vi "remove tag.vi"(8 "error in":errorcluster, 10 "tag":string, 11 "object ref in":T1) -> (0 "error out":errorcluster)   [LabVIEW 2013, in "Shared Memory Editor Node.lvclass"]
doc: "Copyright 2016 National Instruments Corporation\n\nLicensed under the Apache License, Version 2.0 (the \"License\"); you may not use this file except in compliance with the License. You may obtain a copy of the License at http://www.apache.org/licenses/LICENSE-2.0\nUnless required by applicable law or agreed to in writing, software distributed under the License is distributed on an \"AS IS\" BASIS, WITHOUT WARRANTIES OR CONDITIONS OF ANY KIND, either express or implied. See the License for the specific language governing permissions and limitations under the License."
uses:
  Shared Memory Editor Node.lvclass
  <vilib>/NI/DCAF Table API/Table Manager/object ref.ctl
  <vilib>/NI/DCAF/Tag Editor Core/Configuration Editor/Classes/Engine Parent/Engine Parent Editor Node.lvclass
  <vilib>/NI/DCAF/Tag Editor Core/Configuration Editor/Classes/Module editor node/module editor node.lvclass
  module/configuration/Shared Memory Configuration.lvclass
  <vilib>/NI/Configuration Framework/serializable configuration/NISE_CEF_serializable configuration.lvclass/NISE_CEF_serializable configuration.ctl
  <vilib>/Utility/LVClass/Get LV Class Name.vi
  <vilib>/NI/Configuration Framework/error generator/NISE_error generator.vi
  <vilib>/NI/Configuration Framework/serializable configuration/NISE_CEF_serializable configuration.lvclass
  <vilib>/NI/Module Execution Interface/Engine Configuration/engine configuration.lvclass
  <vilib>/NI/DCAF Table API/Table Manager/Table Manager.lvclass
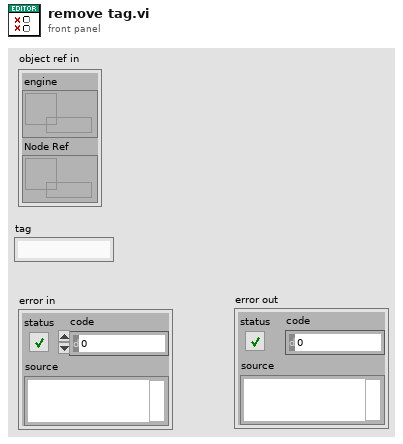
[diagram p1: front panel]
types:
  T1 = typedef "Table Manager.lvlib/Table Manager.lvclass/object ref.ctl" = cluster{"engine":refnum<data-value>, "Node Ref":refnum<data-value>}
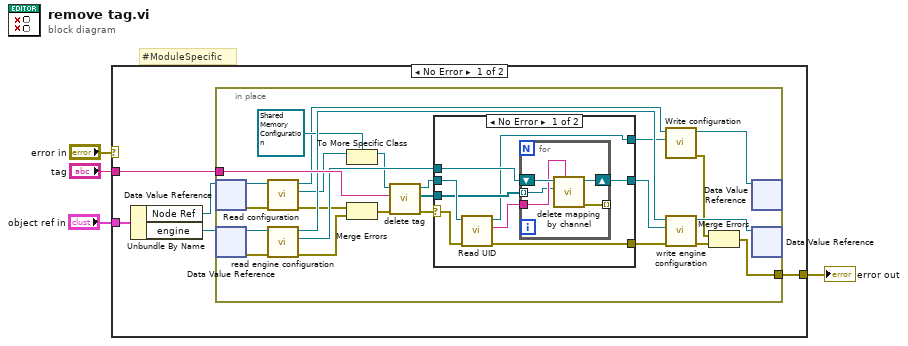
[diagram p0: block diagram]
diagram:
  # "#ModuleSpecific"
  n1 = case shown="No Error" "error in" {
    selector: "error in" -> [_ w51]
    tunnel: [w9 w51] -> w4
    tunnel: "object ref in" -> [w6 _]
    tunnel: "tag" -> [w5 _]
    frame No Error {
      n2 = Unbundle By Name(w6) -> ("Node Ref"=w7:refnum<data-value>, "engine"=w8:refnum<data-value>)
      n3 = in-place {
        in-place-border: [w10] -> w9
        in-place-border: w5 -> [w30]
        n4 = in-place-dvr #1(w7) -> (w29:refnum<class "module editor node.lvclass">, w31:errorcluster)
        n5 = in-place-dvr #2(w8) -> (w33:refnum<class "Engine Parent Editor Node.lvclass">, w32:errorcluster)
        n6 = call-dynamic "Read configuration.vi"("error in"=w31, "NISE_CEF_serializable node in"=w29) -> ("error out"=w15:errorcluster, "configuration"=w17:refnum<class "NISE_CEF_serializable configuration.lvclass">, "NISE_CEF_serializable node out"=w12:refnum<class "module editor node.lvclass">)  [unwired: 7 in]
        n7 = call <vilib>:"read engine configuration.vi"("error in"=w32, "Engine Parent Editor Node in"=w33) -> ("error out"=w24:errorcluster, "engine configuration"=w26:refnum<class "engine configuration.lvclass">, "Engine Parent Editor Node out"=w25:refnum<class "Engine Parent Editor Node.lvclass">)  [unwired: 7 in]
        n8 = To More Specific Class(target class=refnum<class "Shared Memory Configuration.lvclass"> refnum ("tag select  module configuration in"), reference=w17) -> (specific class reference=w16:refnum<class "Shared Memory Configuration.lvclass">)  [unwired: 1 in, 1 out]
        n9 = Merge Errors(w15, w24) -> (w23:errorcluster)
        n10 = call "delete tag.vi"("error in"=w23, "tag name"=w30, "shared memory module configuration"=w16) -> ("error out"=w22:errorcluster, "deleted channels"=w21:refnum<class "TBM channel.lvclass">[], "shared memory module configuration out"=w19:refnum<class "Shared Memory Configuration.lvclass">)  [unwired: 6 in]
        n11 = case shown="No Error" w22 {
          selector: w22 -> [w38 w49]
          tunnel: [w37 w49] -> w20
          tunnel: w19 -> [w40 w48]
          tunnel: w26 -> [w42 w50]
          tunnel: [w41 w50] -> w27
          tunnel: w21 -> [w36 _]
          tunnel: [w35 w48] -> w11
          frame No Error {
            n12 = call <vilib>:"Read UID.vi"("error in"=w38, "configuration in"=w40) -> ("error out"=w37:errorcluster, "instance id"=w39:string, "configuration out"=w35:refnum<class "Shared Memory Configuration.lvclass">)  [unwired: 7 in]
            n13 = for {
              tunnel: w39 -> [w45]
              shift-right: [w46] -> w41
              shift-left: w42 -> [w47]
              tunnel: [w44] -> _ mode=indexing
              tunnel: w36 -> [w43] mode=indexing
              n14 = call <vilib>:"delete mapping by channel.vi"("owner ID"=w45, "channel"=w43, "engine configuration in"=w47) -> ("error out"=w44:errorcluster, "engine configuration out"=w46:refnum<class "engine configuration.lvclass">)  [unwired: 7 in]
            }
          }
          frame Error {
          }
        }
        n15 = call-dynamic "Write configuration.vi"("configuration"=w11, "NISE_CEF_serializable node in"=w12) -> ("error out"=w13:errorcluster, "NISE_CEF_serializable node out"=w28:refnum<class "module editor node.lvclass">)  [unwired: 8 in]
        n16 = call <vilib>:"write engine configuration.vi"("error in"=w20, "engine configuration"=w27, "Engine Parent Editor Node in"=w25) -> ("error out"=w14:errorcluster, "Engine Parent Editor Node out"=w34:refnum<class "Engine Parent Editor Node.lvclass">)  [unwired: 7 in]
        n17 = Merge Errors(w13, w14) -> (w10:errorcluster)
        n18 = in-place-dvr #1(w28) -> ()  [unwired: 2 out]
        n19 = in-place-dvr #2(w34) -> ()  [unwired: 2 out]
      }
    }
    frame Error {
    }
  }
  "error out" <- w4
